vi "TachoInterface.vi"(11 "Called?":bool) -> ()   [LabVIEW 2023]
uses:
  Controls/DisplayQCommand.ctl
  Controls/DisplayMessage.ctl
panel:
  in  "Tacho Interface":bool
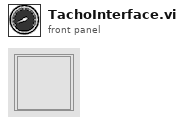
[diagram p1: front panel]
types:
  T1 = enum8{"Enabled", "Disabled", "Disabled and Grayed Out"}
  T2 = typedef "DisplayMessage.ctl" = enum16{"No Message - Ignore", "Display Message", "Set Tab", "Set Status", "Add Error Message", "Clear Error History", "Generate Error", "Set Idling Display", "Set Running Display", "Set Subpanel Output", "Stop"}
  T3 = typedef "DisplayQCommand.ctl" = enum16{"No Command - Error", "Initialise", "Get Q Reference", "Add Item to Bottom", "Add Item to Top", "Flush Q", "Dequeue", "Peek Next Element", "Close"}
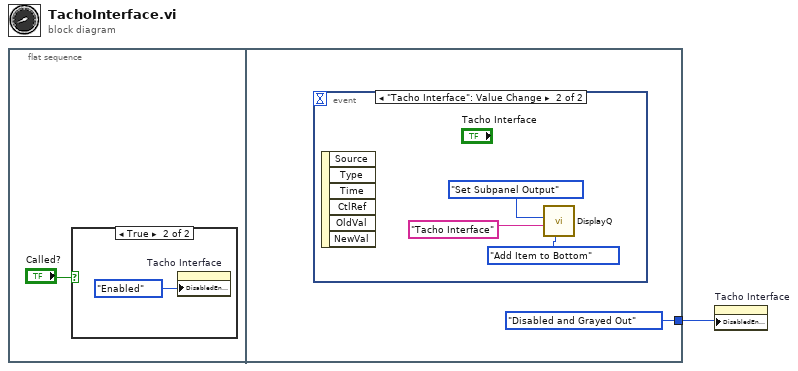
[diagram p0: block diagram]
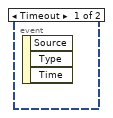
[diagram p3: hidden frame]
diagram:
  n1 = flat-sequence {
    tunnel: [T1."Disabled and Grayed Out" ("Disabled")] -> w1
    frame #0 {
      n2 = case shown="True" "Called?" {
        frame False {
        }
        frame True {
          n3 = property on="Tacho Interface" class="Bool"("DisabledEnum"=T1."Enabled" ("Disabled")) -> ()  [unwired: 2 in, 2 out]
        }
      }
    }
    frame #1 {
      n4 = event shown="[1] \"Tacho Interface\": Value Change" {
        selector: _ -> [_ _]
        dyn-events: _ -> [_ _]
        timeout: _ -> [_ _]
        event Timeout {
          n5 = event-data() -> ()  [unwired: 1 in, 3 out]
        }
        event "Tacho Interface": Value Change {
          n6 = event-data() -> ()  [unwired: 1 in, 6 out]
          n7 = call "DisplayQ.vi"("command"=DisplayQCommand."Add Item to Bottom", "DataIn"="Tacho Interface", "DisplayMessage"=DisplayMessage."Set Subpanel Output") -> ()  [unwired: 2 in, 4 out]
        }
      }
    }
  }
  n8 = property on="Tacho Interface" class="Bool"("DisabledEnum"=w1) -> ()  [unwired: 2 in, 2 out]
